vi "ReadWrite.ProcessData.Write.vi"(7 "error in (no error)":errorcluster, 8 "Offset":i32, 9 "Values":dbl[](array[numeric]), 10 "ReadWrite in":refnum<class "ReadWrite.lvclass">) -> (0 "error out":errorcluster, 3 "ReadWrite out":refnum<class "ReadWrite.lvclass">)   [LabVIEW 2027, in "Data Access Engine.lvlib" / "ReadWrite.lvclass"]
uses:
  ReadWrite.lvclass
  ReadWrite.lvclass/ReadWrite.ctl
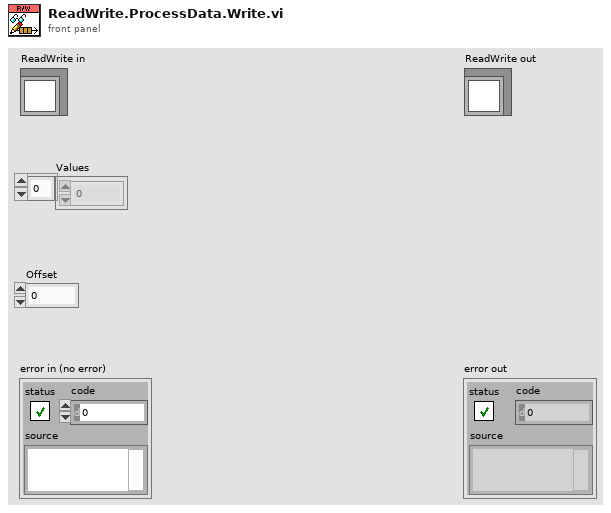
[diagram p1: front panel]
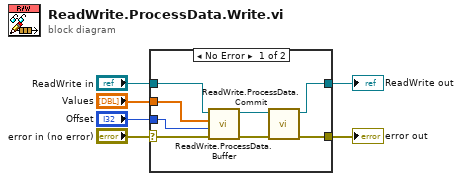
[diagram p0: block diagram]
diagram:
  n1 = case shown="No Error" "error in (no error)" {
    selector: "error in (no error)" -> [w11 w16]
    tunnel: [w8 w16] -> w5
    tunnel: [w7 w15] -> w3
    tunnel: "ReadWrite in" -> [w12 w15]
    tunnel: "Values" -> [w13 _]
    tunnel: "Offset" -> [w14 _]
    frame No Error {
      n2 = call "ReadWrite.ProcessData.Buffer.vi"("error in (no error)"=w11, "Offset"=w14, "Values"=w13, "ReadWrite in"=w12) -> ("error out"=w10:errorcluster, "ReadWrite out"=w9:refnum<class "ReadWrite.lvclass">)  [unwired: 6 in]
      n3 = call "ReadWrite.ProcessData.Commit.vi"("error in (no error)"=w10, "ReadWrite in"=w9) -> ("error out"=w8:errorcluster, "ReadWrite out"=w7:refnum<class "ReadWrite.lvclass">)  [unwired: 8 in]
    }
    frame Error {
    }
  }
  "error out" <- w5
  "ReadWrite out" <- w3
